vi "Lv_BuildPulseGenPico_WithTinyGo.vi"() -> ()   [LabVIEW 2020]
panel:
  in  "output folder":path=path "C:/TEMP"
  in  "Build type":u16(ring) items=["output src", "build uf2", "flash"]
  in  "Tab":T1(tab) caption="Select microcontroller"
  in  "pico_target":string(combo)="pico" caption="target"
  in  "pico_pwm":string(combo)="PWM7" caption="pwm"
  in  "pico_pin":string(combo)="GP15" caption="pin"
  in  "ws-rp2040_target":string(combo)="waveshare-rp2040-zero" caption="target"
  in  "ws-rp2040_pwm":string(combo)="PWM7" caption="pwm"
  in  "ws-rp2040_pin":string(combo)="D14" caption="pin"
  in  "seeed_rp2040_target":string(combo)="xiao-rp2040" caption="target"
  in  "seeed_rp2040_pwm":string(combo)="PWM0" caption="pwm"
  in  "seeed_rp2040_pin":string(combo)="D7" caption="pin"
  out "return code":i32
  out "error out":errorcluster
  out "concatenated string":string
  out "tinygo src string":string
  in  "Freq(Hz)":i32=1000 format="%.0p"
  # "Build Pulse Generator on Raspi-pico or RP2040 microcontroller using tinygo."
  # "1k .. 1M (1k, 2k, 5k 10k, ..  100k,200k,500k, 1M)"
  # "duty 50%\noutput level 3.3V"
  # "output src: tinygo source only\nbuild uf2: tinygo source and build uf2 file.\nflash: tinygo source and build uf2 direct flash\n  to microcontroller."
  # "GP15 (Pin20)"
  # "https://tinygo.org/docs/reference/microcontrollers/pico/"
  # "D14 (Pin 14)"
  # "https://tinygo.org/docs/reference/microcontrollers/waveshare-rp2040-zero/"
  # "D7 (Pin 7)"
  # "https://tinygo.org/docs/reference/microcontrollers/xiao-rp2040/"
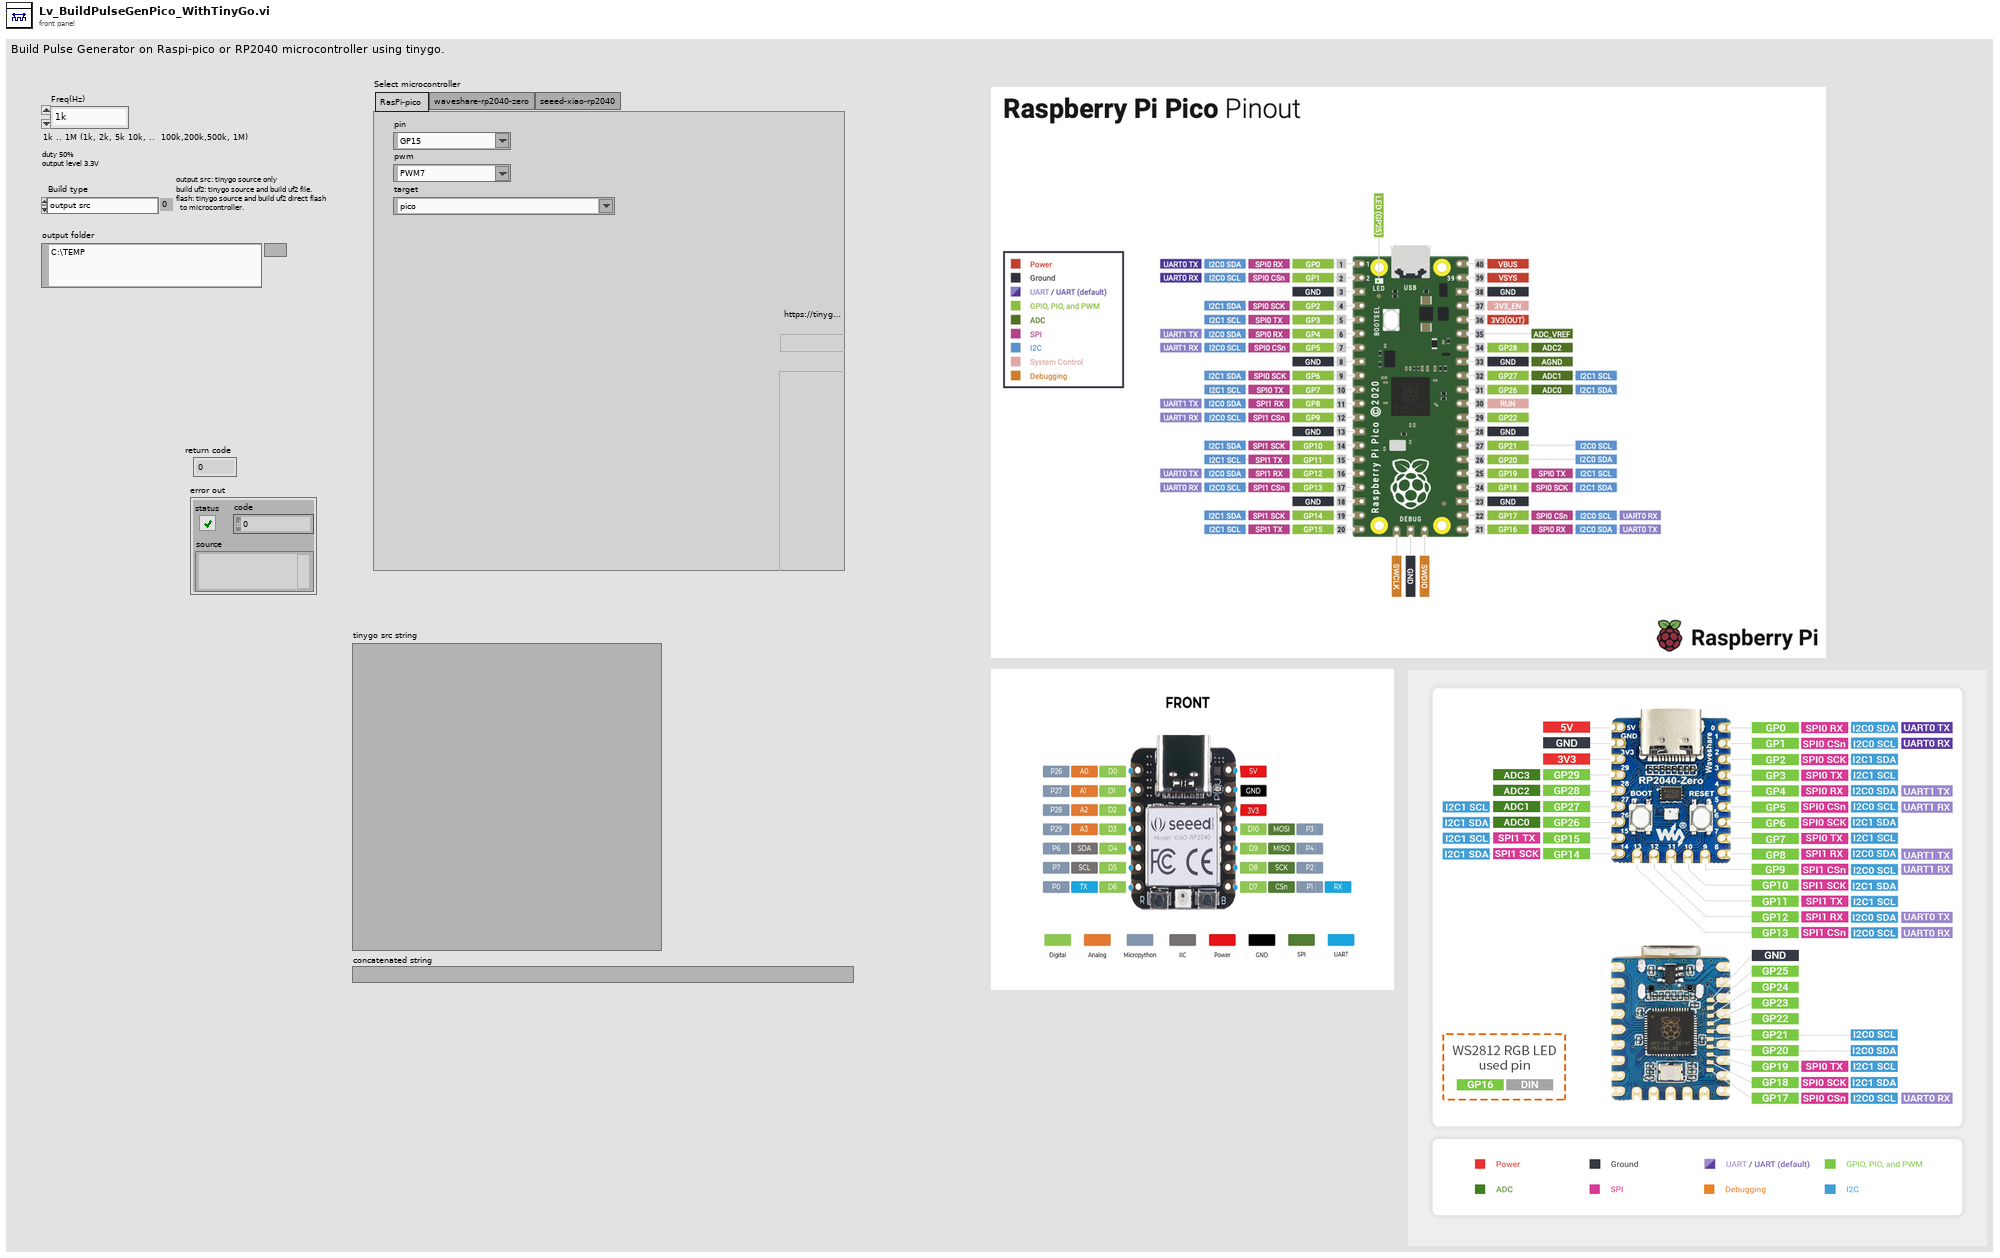
[diagram p1: front panel]
types:
  T1 = enum32{"RasPi-pico", "waveshare-rp2040-zero", "seeed-xiao-rp2040"}
  T2 = enum16{"open", "replace", "create", "open or create", "replace or create", "replace or create with confirmation"}
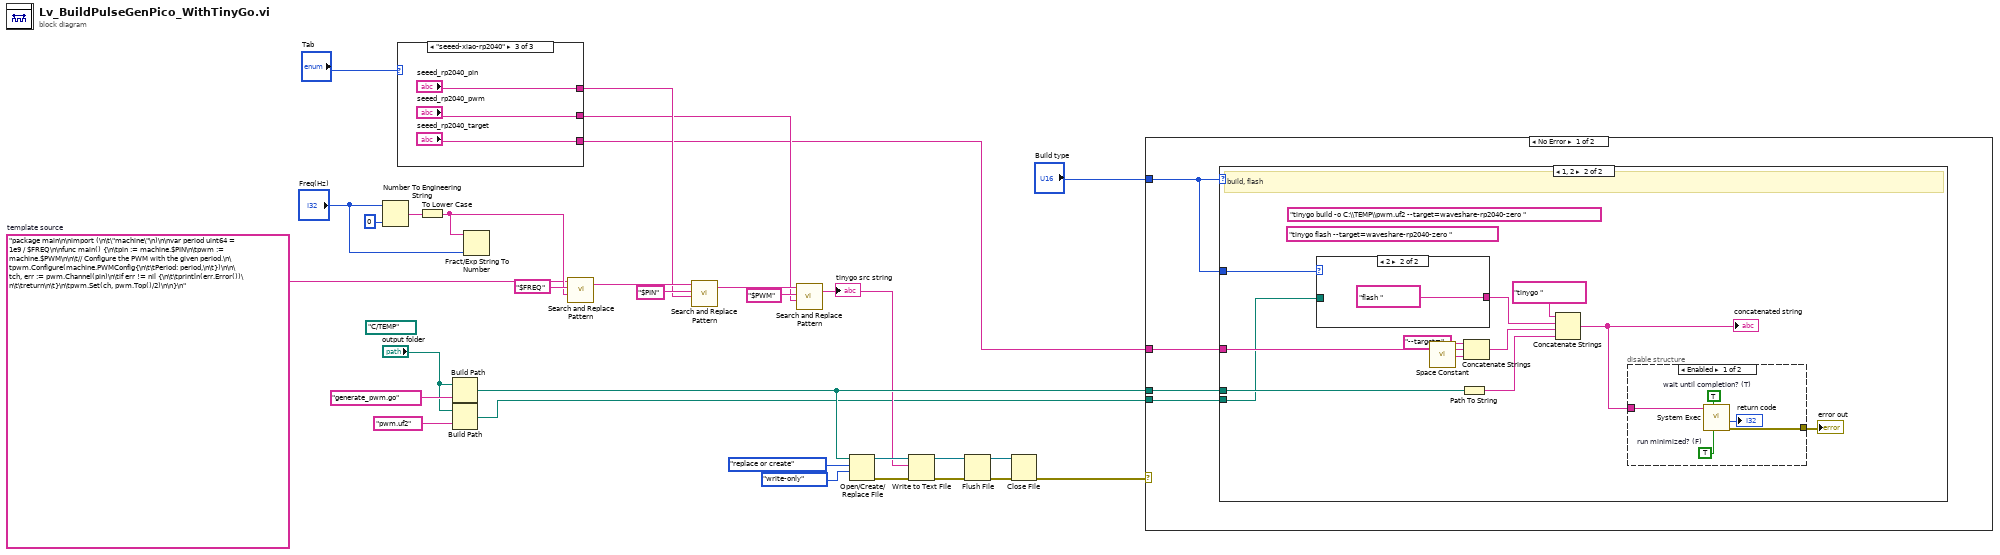
[diagram p0: block diagram]
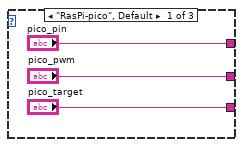
[diagram p2: hidden frame]
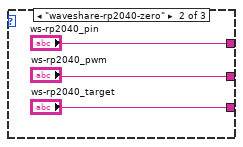
[diagram p3: hidden frame]
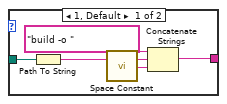
[diagram p5: hidden frame]
diagram:
  (unwired) path "C:/TEMP" ("base path")
  w25 = "package main\n\nimport (\n\t\"machine\"\n)\n\nvar period uint64 = 1e9 / $FREQ\n\nfunc main() {\n\tpin := machine.$PIN\n\tpwm := machine.$PWM\n\n\t// Configure the PWM with the given period.\n\tpwm.Configure(machine.PWMConfig{\n\t\tPeriod: period,\n\t})\n\n\tch, err := pwm.Channel(pin)\n\tif err != nil {\n\t\tprintln(err.Error())\n\t\treturn\n\t}\n\tpwm.Set(ch, pwm.Top()/2)\n\n}\n"  # template source
  n1 = Number To Engineering String(2:i16 0 ("precision (6)"), 4:"Freq(Hz)") -> (0:w30:string)  [unwired: 2 in]
  n2 = case shown="\"seeed-xiao-rp2040\"" "Tab" {
    tunnel: ["pico_pin" "ws-rp2040_pin" "seeed_rp2040_pin"] -> w12
    tunnel: ["pico_pwm" "ws-rp2040_pwm" "seeed_rp2040_pwm"] -> w11
    tunnel: ["pico_target" "ws-rp2040_target" "seeed_rp2040_target"] -> w9
    frame "RasPi-pico", Default {
    }
    frame "waveshare-rp2040-zero" {
    }
    frame "seeed-xiao-rp2040" {
    }
  }
  n3 = To Lower Case(string=w30) -> (all lower case string=w26:string)
  n4 = Build Path(base path="output folder", name or relative path="generate_pwm.go") -> (appended path=w18:path)
  n5 = Build Path(base path="output folder", name or relative path="pwm.uf2") -> (appended path=w2:path)
  n6 = Fract/Exp String To Number(string=w26, default (0 dbl)="Freq(Hz)") -> ()  [unwired: 2 in, 2 out]
  n7 = call <vilib>:"Search and Replace Pattern.vi"("string"=w25, "regular expression (\"\")"="$FREQ" ("regular expression (\"\")"), "replace string (\"\")"=w26) -> ("result string"=w17:string)  [unwired: 2 in, 1 out]
  n8 = call <vilib>:"Search and Replace Pattern.vi"("string"=w17, "regular expression (\"\")"="$PIN" ("regular expression (\"\")"), "replace string (\"\")"=w12) -> ("result string"=w16:string)  [unwired: 2 in, 1 out]
  n9 = call <vilib>:"Search and Replace Pattern.vi"("string"=w16, "regular expression (\"\")"="$PWM" ("regular expression (\"\")"), "replace string (\"\")"=w11) -> ("result string"=w10:string)  [unwired: 2 in, 1 out]
  "tinygo src string" <- w10
  n10 = Open/Create/Replace File(file path (use dialog)=w18, operation (0:open)=T2."replace or create", access (0:read/write)=enum16{"read/write", "read-only", "write-only"}."write-only") -> (refnum out=w24:refnum<file>, error out=w23:errorcluster)  [unwired: 3 in, 1 out]
  n11 = Write to Text File(file (use dialog)=w24, text=w10, error in=w23) -> (refnum out=w21:refnum<file>, error out=w7:errorcluster)  [unwired: 1 in, 1 out]
  n12 = Flush File(refnum=w21, error in=w7) -> (refnum out=w8:refnum<file>, error out=w6:errorcluster)
  n13 = Close File(refnum=w8, error in=w6) -> (error out=w1:errorcluster)  [unwired: 1 out]
  n14 = case shown="No Error" w1 {
    tunnel: w18 -> [w43 _]
    tunnel: w9 -> [w42 _]
    tunnel: "Build type" -> [w41 _]
    tunnel: w2 -> [w40 _]
    frame No Error {
      n15 = case shown="1, 2" w41 {
        tunnel: w43 -> [_ w55]
        tunnel: w42 -> [_ w48]
        tunnel: w41 -> [_ w51]
        tunnel: w40 -> [_ w46]
        frame 0, Default {
          # "output src ony"
        }
        frame 1, 2 {
          (unwired) "tinygo flash --target=waveshare-rp2040-zero "
          (unwired) "tinygo build -o C:\\TEMP\\pwm.uf2 --target=waveshare-rp2040-zero "
          # "build, flash"
          n16 = case shown="2" w51 {
            tunnel: [w56 "flash "] -> w45
            tunnel: w46 -> [w57 _]
            frame 1, Default {
              n17 = Path To String(path=w57) -> (string=w58:string)
              n18 = call <vilib>:"Space Constant.vi"() -> ("String"=w60:string)
              n19 = Concatenate Strings("build -o ", w58, w60) -> (w56:string)
            }
            frame 2 {
            }
          }
          n20 = call <vilib>:"Space Constant.vi"() -> ("String"=w47:string)
          n21 = Path To String(path=w55) -> (string=w54:string)
          n22 = Concatenate Strings("--target=", w48, w47) -> (w44:string)
          n23 = Concatenate Strings("tinygo ", w45, w44, w54) -> (w53:string)
          "concatenated string" <- w53
          n24 = disable-structure shown="Enabled" {
            disable-tunnel: w53 -> [w66 _]
            disable-tunnel: [w65 _] -> w52
            frame Enabled {
              w62 = TRUE  # wait until completion? (T)
              w63 = TRUE  # run minimized? (F)
              n25 = call <vilib>:"System Exec.vi"("run minimized? (F)"=w63, "wait until completion? (T)"=w62, "command line"=w66) -> ("error out"=w65:errorcluster, "return code"=→"return code":i32)  [unwired: 5 in, 2 out]
            }
            frame Disabled {
            }
          }
          "error out" <- w52
        }
      }
    }
    frame Error {
    }
  }
